vi "monochromatorCommandGetUnits.vi"(8 "error in":errorcluster, 11 "monochromator":refnum<k24>) -> (0 "error out":errorcluster, 2 "units":string, 3 "monochromator":refnum<k24>)   [LabVIEW 2009]
doc: "Get Wavelength units used\nReturn string"
uses:
  C:/Users/anderson.chen/Desktop/Software Development/Cornerstone Series API (LV9)/Cornerstone DLL/Cornerstone.dll
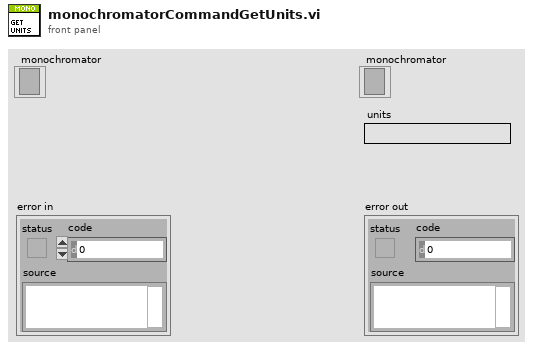
[diagram p1: front panel]
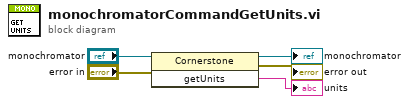
[diagram p0: block diagram]
diagram:
  n1 = invoke class="Cornerstone" method="getUnits"(reference="monochromator", error in="error in") -> (reference out=→"monochromator":refnum<k24>, error out=→"error out":errorcluster, "getUnits"=→"units":string)  [unwired: 1 in]
